vi "Configure Marker.vi"(0 "VISA resource name":refnum<visa-resource-name>, 1 "Delta Reference Marker (0: Marker0)":u16(ring) items=["Marker0", "Marker1", "Marker2", "Marker3", "Marker4", "Marker5", "Marker6", "Marker7", "Marker8", "Marker9", "Marker10", "Marker11", "Marker12", "Marker13", "Marker14", "Marker15", "Marker16", "Marker17", "Marker18", "Marker19"], 2 "Marker Mode (0: Frequency)":u16(ring) items=["Frequency", "Delta"], 5 "Marker (0: Marker0)":u16(ring) items=["Marker0", "Marker1", "Marker2", "Marker3", "Marker4", "Marker5", "Marker6", "Marker7", "Marker8", "Marker9", "Marker10", "Marker11", "Marker12", "Marker13", "Marker14", "Marker15", "Marker16", "Marker17", "Marker18", "Marker19"], 7 "Enable Marker (F:Disable)":bool, 9 "Marker Frequency (528 MHz)":dbl=528000000.0, 11 "error in (no error)":errorcluster, 12 "Enable Marker Amplitude (F:Disable)":bool, 13 "Marker Amplitude (2 dB)":dbl=2.0) -> (4 "VISA resource name out":refnum<visa-resource-name>, 15 "error out":errorcluster)   [LabVIEW 2012, in "Agilent PSG MXG Series.lvlib"]
doc: "Configures marker mode, marker reference, marker state, marker frequency and marker amplitude.\n\n<B>Notes:</B>\n(1) This VI is valid only in E8247C, E8257C, E8267C, E8257D, E8267D, N5183A, N5172B, N5182B.\n\n(2) For E8247C, E8257C, E8267C, E8257D, E8267D, this VI is valid only when the instrument installs <B>Option 007</B> (Analog ramp sweep)."
uses:
  <instrlib>/Agilent PSG MXG Series/Agilent PSG MXG Series.lvlib
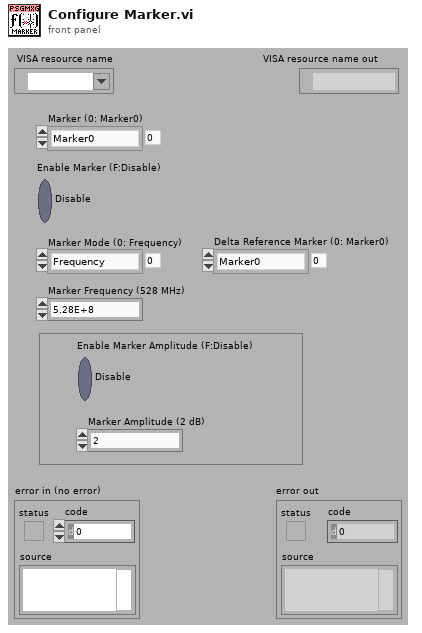
[diagram p1: front panel]
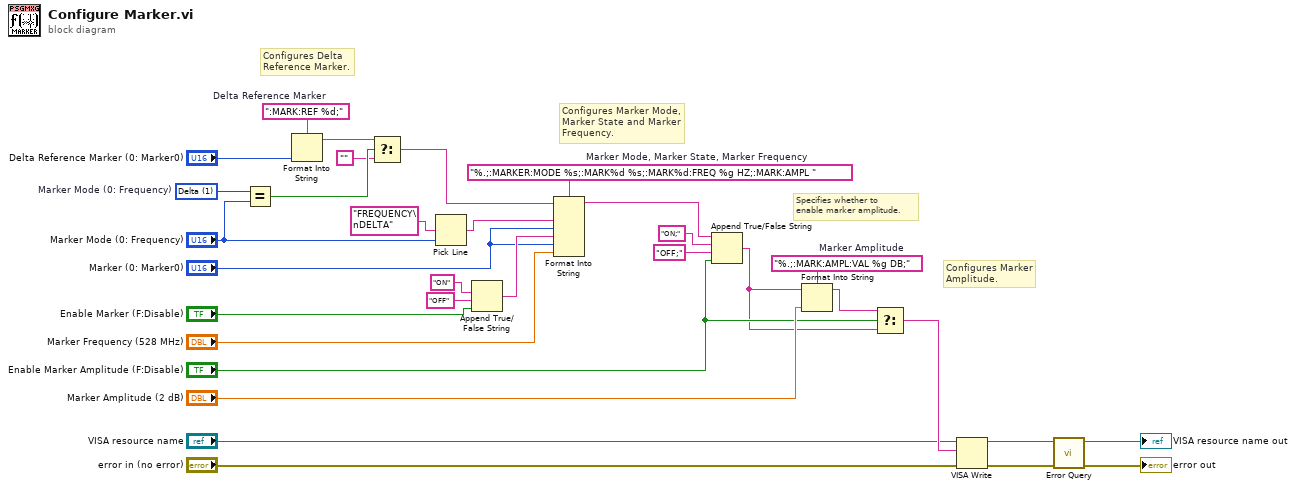
[diagram p0: block diagram]
diagram:
  w20 = ":MARK:REF %d;"  # Delta Reference Marker
  w14 = u16 1 items=["Frequency", "Delta"]  # Marker Mode (0: Frequency)
  w28 = "%.;:MARK:AMPL:VAL %g DB;"  # Marker Amplitude
  w31 = "%.;:MARKER:MODE %s;:MARK%d %s;:MARK%d:FREQ %g HZ;:MARK:AMPL "  # Marker Mode, Marker State, Marker Frequency
  # "Configures Marker\nAmplitude."
  # "Configures Marker Mode,\nMarker State and Marker\nFrequency."
  # "Configures Delta\nReference Marker."
  # "Specifies whether to\nenable marker amplitude."
  n1 = Equal?(x=w14, y="Marker Mode (0: Frequency)") -> (x = y?=w17:bool)
  n2 = Format Into String(format string=w20, "Delta Reference Marker (0: Marker0)") -> (resulting string=w18:string)  [unwired: 2 in, 1 out]
  n3 = Select(t=w18, s=w17, f="") -> (s? t:f=w12:string)
  n4 = Pick Line(multi-line string="FREQUENCY\nDELTA", line index="Marker Mode (0: Frequency)") -> (output string=w15:string)  [unwired: 1 out]
  n5 = Append True/False String(1:"Enable Marker (F:Disable)", 2:"OFF" ("false string"), 3:"ON" ("true string")) -> (0:w11:string)  [unwired: 1 out]
  n6 = Format Into String(format string=w31, initial string=w12, w15, "Marker (0: Marker0)", w11, "Marker (0: Marker0)", "Marker Frequency (528 MHz)") -> (resulting string=w5:string)  [unwired: 1 in, 1 out]
  n7 = Append True/False String(1:"Enable Marker Amplitude (F:Disable)", 2:"OFF;" ("false string"), 3:"ON;" ("true string"), 4:w5) -> (0:w24:string)
  n8 = Format Into String(format string=w28, initial string=w24, "Marker Amplitude (2 dB)") -> (resulting string=w25:string)  [unwired: 1 in, 1 out]
  n9 = Select(t=w25, s="Enable Marker Amplitude (F:Disable)", f=w24) -> (s? t:f=w23:string)
  n10 = VISA Write(VISA resource name="VISA resource name", write buffer=w23, error in (no error)="error in (no error)") -> (VISA resource name out=w22:refnum<visa-resource-name>, error out=w21:errorcluster)  [unwired: 1 out]
  n11 = call <instrlib>:"Error Query.vi"("error in (no error)"=w21, "VISA resource name"=w22) -> ("error out"=→"error out":errorcluster, "VISA resource name out"=→"VISA resource name out":refnum<visa-resource-name>)  [unwired: 8 out]
